vi "Get Power Measurement.vi"(6 "Cal Route":string[](array[string]), 7 "Cal?":bool, 8 "error in (no error)":errorcluster, 9 "Rnd?":bool, 10 "Frequency":dbl=1000000000.0, 11 "VISA Refnum in":refnum<visa-resource-name>) -> (0 "error out":errorcluster, 2 "Measurement":dbl, 3 "VISA Refnum out":refnum<visa-resource-name>)   [LabVIEW 2015]
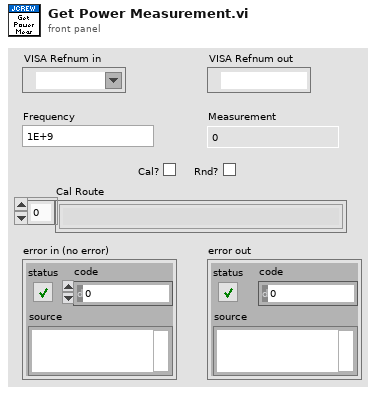
[diagram p1: front panel]
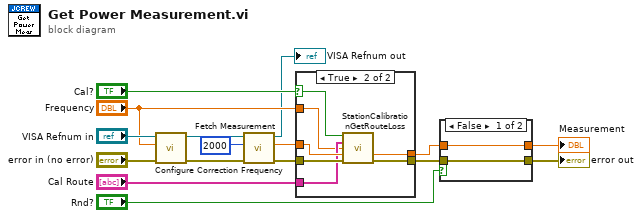
[diagram p0: block diagram]
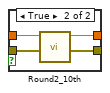
[diagram p2: hidden frame]
diagram:
  n1 = call <instrlib>:"Configure Correction Frequency.vi"("error in (no error)"="error in (no error)", "Frequency (5E+7 Hz)"="Frequency", "VISA resource name"="VISA Refnum in") -> ("error out"=w3:errorcluster, "VISA resource name out"=w6:refnum<visa-resource-name>)  [unwired: 7 in]
  n2 = call <instrlib>:"Fetch Measurement.vi"("error in (no error)"=w3, "Timeout (10000 ms)"=u32 2000, "VISA resource name"=w6) -> ("error out"=w4:errorcluster, "Measurement"=w5:dbl, "VISA resource name out"=→"VISA Refnum out":refnum<visa-resource-name>)  [unwired: 6 out]
  n3 = case shown="True" "Cal?" {
    selector: "Cal?" -> [_ w19]
    tunnel: [w17 w25] -> w11
    tunnel: [w18 w20] -> w9
    tunnel: w4 -> [w18 w24]
    tunnel: w5 -> [w17 w23]
    tunnel: "Cal Route" -> [_ w22]
    tunnel: "Frequency" -> [_ w21]
    frame False {
    }
    frame True {
      n4 = call "StationCalibrationGetRouteLoss.vi"("Calibration Enabled"=w19, "Route Names"=w22, "Frequency"=w21, "Power Level"=w23, "error in (no error)"=w24) -> ("Adjusted Power Level"=w25:dbl, "error out"=w20:errorcluster)  [unwired: 7 in, 2 out]
    }
  }
  n5 = case shown="False" "Rnd?" {
    tunnel: w11 -> [w27 w30]
    tunnel: [w27 w29] -> w10
    tunnel: [w26 w28] -> w8
    tunnel: w9 -> [w26 w28]
    frame False {
    }
    frame True {
      n6 = call "Round2_10th.vi"("Newman"=w30) -> ("Newmout"=w29:dbl)  [unwired: 10 in]
    }
  }
  "Measurement" <- w10
  "error out" <- w8
